vi "Finish.vi"   [LabVIEW 2019]
doc: "This VI is called just before exiting. It is expected to close I/O refnum, save collected data, etc."
uses:
  <vilib>/Rock Robotics/WPI/Utilities/WPI_GetSetVariantRefNum.vi
types:
  T1 = typedef "WPI_JoystickDevRef.ctl" = cluster{"Device":T2}
  T2 = typedef "WPI_JoystickDeviceEnum.ctl" = enum16{"USB 0", "USB 1", "USB 2", "USB 3", "USB 4", "USB 5"}
  T3 = typedef "WPI_RobotDriveDevRef.ctl" = cluster{"DevStatus":errorcluster, "Motors[]":T4[], "Square Inputs":bool, "Max Output":dbl}
  T4 = typedef "WPI_MotorControlDeviceRef.ctl" = cluster{"DeviceStatus":errorcluster, "Type":T5, "PWM":cluster{"PWM Channel":T6, "DeadBand":T7}, "CAN":cluster{"Device Number":u8, "SetOutput VI Ref":variant, "GetOutput VI Ref":variant, "Enable VI Ref":variant, "Disable VI Ref":variant, "Data":variant}, "Invert":bool, "DIO PWM":cluster{"PWM \"Enable\" Channel":T6, "DIOChannel":T8, "PWM Rate":dbl}}
  T5 = typedef "WPI_MotorControlType.ctl" = enum16{"PWM", "CAN", "DIO PWM"}
  T6 = typedef "FPGA_DIOPWMChannel.ctl" = enum8{"PWM 0", "PWM 1", "PWM 2", "PWM 3", "PWM 4", "PWM 5", "PWM 6", "PWM 7", "PWM 8", "PWM 9", "PWM MXP 0", "PWM MXP 1", "PWM MXP 2", "PWM MXP 3", "PWM MXP 4", "PWM MXP 5", "PWM MXP 6", "PWM MXP 7", "PWM MXP 8", "PWM MXP 9", "Invalid"}
  T7 = typedef "WPI_PWMDeadband.ctl" = cluster{"Name":string, "maxPositivePwm":i32, "minPositivePwm":i32, "centerPwm":i32, "maxNegativePwm":i32, "minNegativePwm":i32, "angularRange":u16}
  T8 = typedef "FPGA_DIOChannel.ctl" = enum8{"DIO 0", "DIO 1", "DIO 2", "DIO 3", "DIO 4", "DIO 5", "DIO 6", "DIO 7", "DIO 8", "DIO 9", "DIO MXP 0", "DIO MXP 1", "DIO MXP 2", "DIO MXP 3", "DIO MXP 4", "DIO MXP 5", "DIO MXP 6", "DIO MXP 7", "DIO MXP 8", "DIO MXP 9", "DIO MXP 10", "DIO MXP 11", "DIO MXP 12", "DIO MXP 13", "DIO MXP 14", "DIO MXP 15", "SPI Port CS1", "SPI Port CS2", "SPI Port CS3", "SPI Port MISO", "SPI Port MOSI", "Invalid"}
  T9 = typedef "WPI_SolenoidDevRef.ctl" = cluster{"DevStatus":errorcluster, "Pneumatics Control Module":u8, "Forward Solenoid Channel":T10, "Reverse Solenoid Channel":T10}
  T10 = typedef "WPI_SolenoidChannel.ctl" = enum8{"Solenoid 0", "Solenoid 1", "Solenoid 2", "Solenoid 3", "Solenoid 4", "Solenoid 5", "Solenoid 6", "Solenoid 7", "Invalid"}
  T11 = typedef "WPI_SwitchDevRef.ctl" = cluster{"DevStatus":errorcluster, "DIO Channel":T8, "CntIndex":T12, "Normally Closed":bool}
  T12 = typedef "FPGA_CounterCtrSystemIndex.ctl" = enum8{"Ctr 0", "Ctr 1", "Ctr 2", "Ctr 3", "Ctr 4", "Ctr 5", "Ctr 6", "Ctr 7", "Invalid"}
  T13 = typedef "WPI_EncoderDevRef.ctl" = cluster{"DevStatus":errorcluster, "EncoderIndex":T14, "CounterIndex":T12, "DistancePerCount":dbl, "Decoding Type":T15}
  T14 = typedef "FPGA_EncoderIdx.ctl" = enum8{"Enc 0", "Enc 1", "Enc 2", "Enc 3", "Enc 4", "Enc 5", "Enc 6", "Enc 7", "Invalid"}
  T15 = typedef "WPI_EncoderType.ctl" = enum16{"1x", "2x", "4x"}
  T16 = typedef "WPI_CompressorDevRef.ctl" = cluster{"DevStatus":errorcluster, "Pneumatics Control Module":u8}
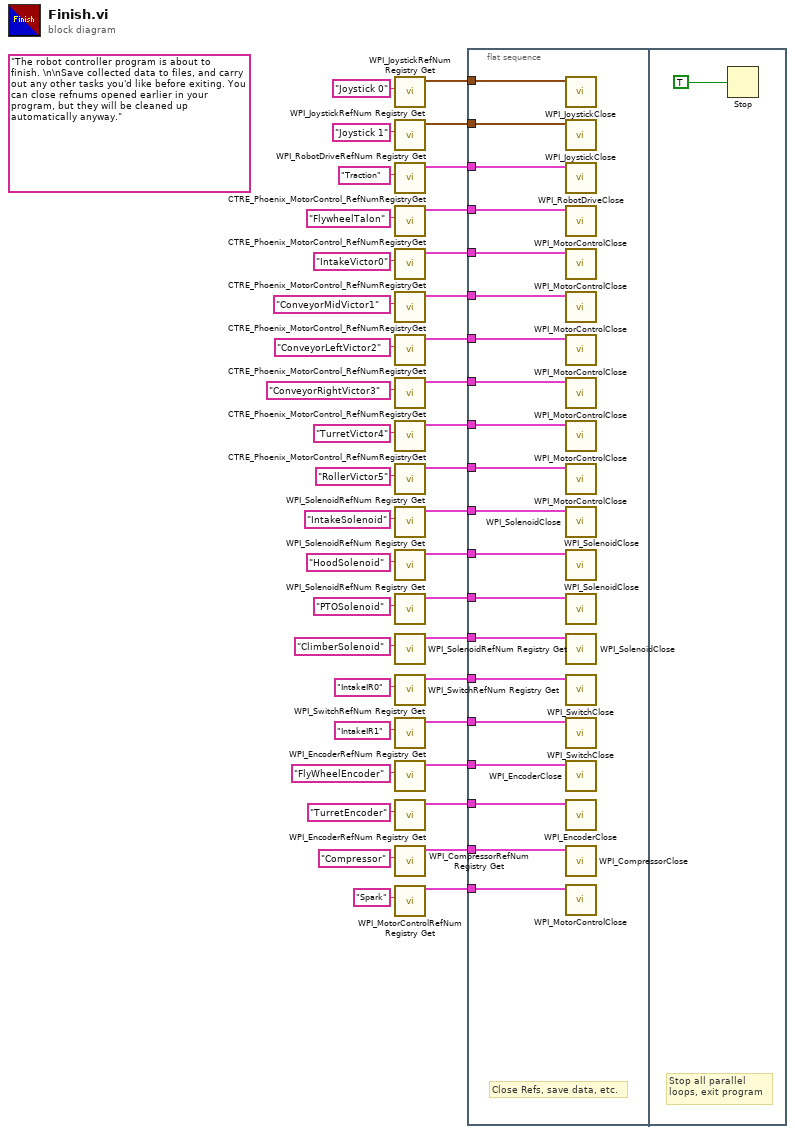
[diagram p0: block diagram]
diagram:
  (unwired) "The robot controller program is about to finish. \n\nSave collected data to files, and carry out any other tasks you'd like before exiting. You can close refnums opened earlier in your program, but they will be cleaned up automatically anyway."
  n1 = call <vilib>:"WPI_JoystickRefNum Registry Get.vi"("refnum name"="Joystick 0") -> ("JoystickDevRef"=w37:T1)  [unwired: 1 in, 9 out]
  n2 = call <vilib>:"WPI_JoystickRefNum Registry Get.vi"("refnum name"="Joystick 1") -> ("JoystickDevRef"=w36:T1)  [unwired: 1 in, 9 out]
  n3 = call <vilib>:"WPI_RobotDriveRefNum Registry Get.vi"("refnum name"="Traction") -> ("RobotDriveDevRef"=w38:T3)  [unwired: 1 in, 9 out]
  n4 = call <vilib>:"CTRE_Phoenix_MotorControl_RefNumRegistryGet.vi"("refnum name"="FlywheelTalon") -> ("PhoenixMotorControlDevRef"=w32:T4)  [unwired: 9 in, 1 out]
  n5 = call <vilib>:"CTRE_Phoenix_MotorControl_RefNumRegistryGet.vi"("refnum name"="IntakeVictor0") -> ("PhoenixMotorControlDevRef"=w23:T4)  [unwired: 9 in, 1 out]
  n6 = call <vilib>:"CTRE_Phoenix_MotorControl_RefNumRegistryGet.vi"("refnum name"="ConveyorMidVictor1") -> ("PhoenixMotorControlDevRef"=w24:T4)  [unwired: 9 in, 1 out]
  n7 = call <vilib>:"CTRE_Phoenix_MotorControl_RefNumRegistryGet.vi"("refnum name"="ConveyorLeftVictor2") -> ("PhoenixMotorControlDevRef"=w25:T4)  [unwired: 9 in, 1 out]
  n8 = call <vilib>:"CTRE_Phoenix_MotorControl_RefNumRegistryGet.vi"("refnum name"="ConveyorRightVictor3") -> ("PhoenixMotorControlDevRef"=w26:T4)  [unwired: 9 in, 1 out]
  n9 = call <vilib>:"CTRE_Phoenix_MotorControl_RefNumRegistryGet.vi"("refnum name"="TurretVictor4") -> ("PhoenixMotorControlDevRef"=w27:T4)  [unwired: 9 in, 1 out]
  n10 = call <vilib>:"CTRE_Phoenix_MotorControl_RefNumRegistryGet.vi"("refnum name"="RollerVictor5") -> ("PhoenixMotorControlDevRef"=w14:T4)  [unwired: 9 in, 1 out]
  n11 = call <vilib>:"WPI_SolenoidRefNum Registry Get.vi"("refnum name"="IntakeSolenoid") -> ("SolenoidDevRef"=w18:T9)  [unwired: 9 in, 1 out]
  n12 = call <vilib>:"WPI_SolenoidRefNum Registry Get.vi"("refnum name"="HoodSolenoid") -> ("SolenoidDevRef"=w17:T9)  [unwired: 9 in, 1 out]
  n13 = call <vilib>:"WPI_SolenoidRefNum Registry Get.vi"("refnum name"="PTOSolenoid") -> ("SolenoidDevRef"=w4:T9)  [unwired: 9 in, 1 out]
  n14 = call <vilib>:"WPI_SolenoidRefNum Registry Get.vi"("refnum name"="ClimberSolenoid") -> ("SolenoidDevRef"=w16:T9)  [unwired: 9 in, 1 out]
  n15 = call <vilib>:"WPI_SwitchRefNum Registry Get.vi"("refnum name"="IntakeIR0") -> ("SwitchDevRef"=w12:T11)  [unwired: 9 in, 1 out]
  n16 = call <vilib>:"WPI_SwitchRefNum Registry Get.vi"("refnum name"="IntakeIR1") -> ("SwitchDevRef"=w11:T11)  [unwired: 9 in, 1 out]
  n17 = call <vilib>:"WPI_EncoderRefNum Registry Get.vi"("refnum name"="FlyWheelEncoder") -> ("EncoderDevRef"=w35:T13)  [unwired: 9 in, 1 out]
  n18 = call <vilib>:"WPI_EncoderRefNum Registry Get.vi"("refnum name"="TurretEncoder") -> ("EncoderDevRef"=w1:T13)  [unwired: 9 in, 1 out]
  n19 = call <vilib>:"WPI_CompressorRefNum Registry Get.vi"("refnum name"="Compressor") -> ("CompressorDevRef"=w6:T16)  [unwired: 9 in, 1 out]
  n20 = call <vilib>:"WPI_MotorControlRefNum Registry Get.vi"("refnum name"="Spark") -> ("MotorControlDevRef"=w8:T4)  [unwired: 9 in, 1 out]
  n21 = flat-sequence {
    tunnel: w38 -> [w60]
    tunnel: w37 -> [w59]
    tunnel: w36 -> [w58]
    tunnel: w35 -> [w57]
    tunnel: w32 -> [w56]
    tunnel: w27 -> [w55]
    tunnel: w26 -> [w54]
    tunnel: w25 -> [w53]
    tunnel: w24 -> [w52]
    tunnel: w23 -> [w51]
    tunnel: w18 -> [w50]
    tunnel: w17 -> [w49]
    tunnel: w16 -> [w48]
    tunnel: w14 -> [w47]
    tunnel: w12 -> [w46]
    tunnel: w11 -> [w45]
    tunnel: w8 -> [w44]
    tunnel: w6 -> [w43]
    tunnel: w4 -> [w42]
    tunnel: w1 -> [w41]
    frame #0 {
      # "Close Refs, save data, etc."
      n22 = call <vilib>:"WPI_JoystickClose.vi"("JoystickDevRef"=w59) -> ()  [unwired: 11 out]
      n23 = call <vilib>:"WPI_JoystickClose.vi"("JoystickDevRef"=w58) -> ()  [unwired: 11 out]
      n24 = call <vilib>:"WPI_RobotDriveClose.vi"("RobotDriveDevRef"=w60) -> ()  [unwired: 1 in, 10 out]
      n25 = call <vilib>:"WPI_MotorControlClose.vi"("MotorControlDevRef"=w56) -> ()  [unwired: 10 in, 1 out]
      n26 = call <vilib>:"WPI_MotorControlClose.vi"("MotorControlDevRef"=w51) -> ()  [unwired: 10 in, 1 out]
      n27 = call <vilib>:"WPI_MotorControlClose.vi"("MotorControlDevRef"=w52) -> ()  [unwired: 10 in, 1 out]
      n28 = call <vilib>:"WPI_MotorControlClose.vi"("MotorControlDevRef"=w53) -> ()  [unwired: 10 in, 1 out]
      n29 = call <vilib>:"WPI_MotorControlClose.vi"("MotorControlDevRef"=w54) -> ()  [unwired: 10 in, 1 out]
      n30 = call <vilib>:"WPI_MotorControlClose.vi"("MotorControlDevRef"=w55) -> ()  [unwired: 10 in, 1 out]
      n31 = call <vilib>:"WPI_MotorControlClose.vi"("MotorControlDevRef"=w47) -> ()  [unwired: 10 in, 1 out]
      n32 = call <vilib>:"WPI_SolenoidClose.vi"("SolenoidDevRef"=w50) -> ()  [unwired: 10 in, 1 out]
      n33 = call <vilib>:"WPI_SolenoidClose.vi"("SolenoidDevRef"=w49) -> ()  [unwired: 10 in, 1 out]
      n34 = call <vilib>:"WPI_SolenoidClose.vi"("SolenoidDevRef"=w42) -> ()  [unwired: 10 in, 1 out]
      n35 = call <vilib>:"WPI_SolenoidClose.vi"("SolenoidDevRef"=w48) -> ()  [unwired: 10 in, 1 out]
      n36 = call <vilib>:"WPI_SwitchClose.vi"("SwitchDevRef"=w46) -> ()  [unwired: 10 in, 1 out]
      n37 = call <vilib>:"WPI_SwitchClose.vi"("SwitchDevRef"=w45) -> ()  [unwired: 10 in, 1 out]
      n38 = call <vilib>:"WPI_EncoderClose.vi"("EncoderDevRef"=w57) -> ()  [unwired: 10 in, 1 out]
      n39 = call <vilib>:"WPI_EncoderClose.vi"("EncoderDevRef"=w41) -> ()  [unwired: 10 in, 1 out]
      n40 = call <vilib>:"WPI_CompressorClose.vi"("CompressorDevRef"=w43) -> ()  [unwired: 10 in, 1 out]
      n41 = call <vilib>:"WPI_MotorControlClose.vi"("MotorControlDevRef"=w44) -> ()  [unwired: 10 in, 1 out]
    }
    frame #1 {
      # "Stop all parallel\nloops, exit program"
      n42 = Stop(stop? (T)=TRUE ("Quit")) -> ()
    }
  }
